vi "FTW-Supervisor-SerializeEvent.vi"(0 "Event Type":string, 5 "Event Data":string, 7 "Source (unwired for call chain, Empty to omit)":string="CallChain", 11 "Error to Log":errorcluster) -> (4 "Serialized Event":string)   [LabVIEW 2014, in "FTW-Supervisor-Connector.lvclass"]
uses:
  FTW-Supervisor-Connector.lvclass
  time/FTW-Time-DisplayFormat-Timestamp.ctl
panel:
  # "Inputs"
  # "Outputs"
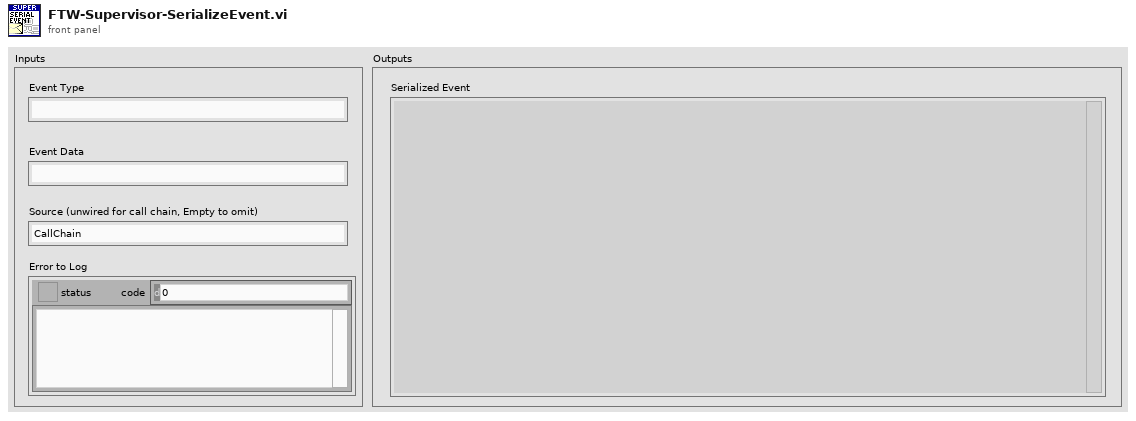
[diagram p1: front panel]
types:
  T1 = typedef "FTW-Time-DisplayFormat-Timestamp.ctl" = enum16{"YYYY-MM-DDT00:00:00.000Z (ISO-8601)", "YYYY-MM-DDT00-00-00Z (Simple ISO-8601)", "YYYY-MM-DD"}
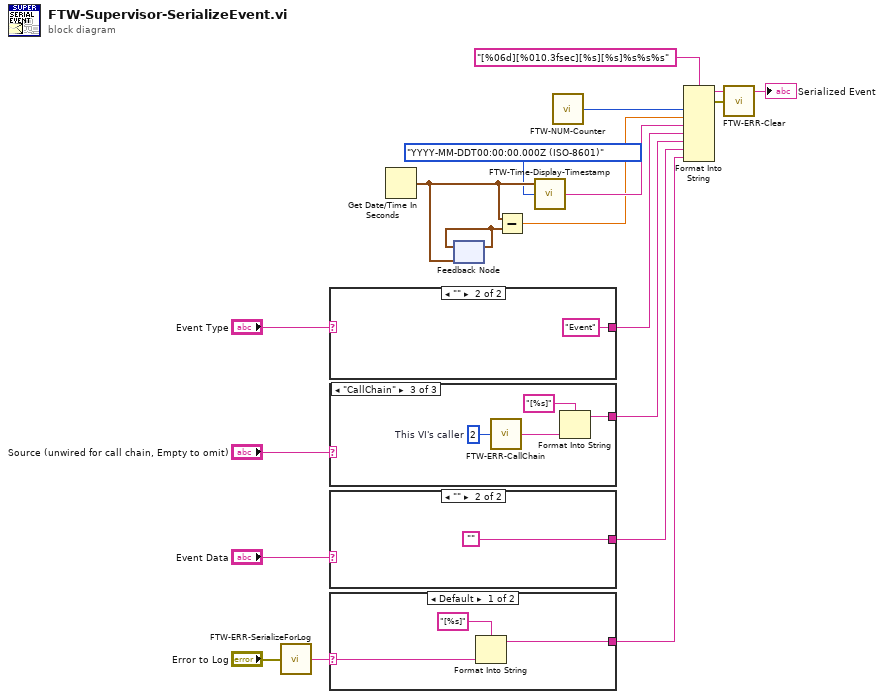
[diagram p0: block diagram]
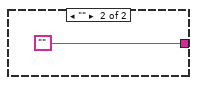
[diagram p2: hidden frame]
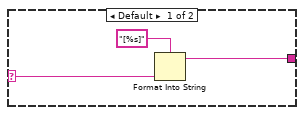
[diagram p4: hidden frame]
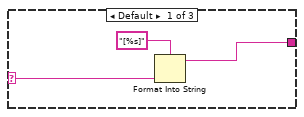
[diagram p5: hidden frame]
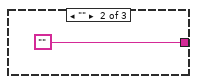
[diagram p6: hidden frame]
diagram:
  n1 = call "FTW-ERR-SerializeForLog.vi"("error in"="Error to Log") -> ("Serialized Error"=w2:string)
  n2 = case shown="\"\"" "Event Type" {
    selector: "Event Type" -> [w19 _]
    tunnel: [w19 "Event"] -> w11
    frame Default {
    }
    frame "" {
    }
  }
  n3 = case shown="\"CallChain\"" "Source (unwired for call chain, Empty to omit)" {
    selector: "Source (unwired for call chain, Empty to omit)" -> [w22 _ _]
    tunnel: [w21 "" w27] -> w13
    frame Default {
      n4 = Format Into String(format string="[%s]", w22) -> (resulting string=w21:string)  [unwired: 2 in, 1 out]
    }
    frame "" {
    }
    frame "CallChain" {
      w26 = 2  # This VI's caller
      n5 = call "FTW-ERR-CallChain.vi"("Levels to exclude (1=This VI's caller)"=w26) -> ("Call Chain"=w25:string)
      n6 = Format Into String(format string="[%s]", w25) -> (resulting string=w27:string)  [unwired: 2 in, 1 out]
    }
  }
  n7 = case shown="\"\"" "Event Data" {
    selector: "Event Data" -> [w31 _]
    tunnel: [w30 ""] -> w14
    frame Default {
      n8 = Format Into String(format string="[%s]", w31) -> (resulting string=w30:string)  [unwired: 2 in, 1 out]
    }
    frame "" {
    }
  }
  n9 = case shown="Default" w2 {
    selector: w2 -> [w35 _]
    tunnel: [w34 ""] -> w1
    frame Default {
      n10 = Format Into String(format string="[%s]", w35) -> (resulting string=w34:string)  [unwired: 2 in, 1 out]
    }
    frame "" {
    }
  }
  n11 = Get Date/Time In Seconds() -> (seconds since 1Jan1904=w4:timestamp)
  n12 = feedback #1(w4) -> (w10:timestamp)
  n13 = feedback-in #1(w10) -> ()
  n14 = Subtract(x=w4, y=w10) -> (x-y=w7:dbl)
  n15 = call "FTW-Time-Display-Timestamp.vi"("Format"=FTW-Time-DisplayFormat-Timestamp."YYYY-MM-DDT00:00:00.000Z (ISO-8601)", "Timestamp (unwired for current time)"=w4) -> ("Formatted Timestamp"=w8:string)  [unwired: 2 in]
  n16 = call "FTW-NUM-Counter.vi"() -> ("Counter"=w5:i32)  [unwired: 1 in]
  n17 = Format Into String(format string="[%06d][%010.3fsec][%s][%s]%s%s%s", w5, w7, w8, w11, w13, w14, w1) -> (resulting string=→"Serialized Event":string, error out=w6:errorcluster)  [unwired: 2 in]
  n18 = call "FTW-ERR-Clear.vi"("error to snuff"=w6) -> ()  [unwired: 1 out]
